vi "Channel Loop.vi"(6 "Event Based?":bool, 7 "Rate":i32=200, 8 "Index":i32, 9 "Waveform Queue":refnum<queue>, 10 "Close Event":refnum<user-event>, 11 "Channel":tag) -> (0 "error out":errorcluster)   [LabVIEW 2020]
uses:
  <vilib>/DAQmx/read.llb/DAQmx Read (Analog Wfm 1Chan NSamp).vi
  <vilib>/DAQmx/create/channels.llb/DAQmx Create Channel (AI-Voltage-Basic).vi
  <vilib>/DAQmx/configure/timing.llb/DAQmx Timing (Sample Clock).vi
  <vilib>/DAQmx/miscellaneous.llb/DAQmx Fill In Error Info.vi
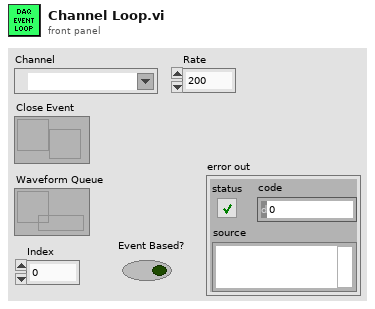
[diagram p1: front panel]
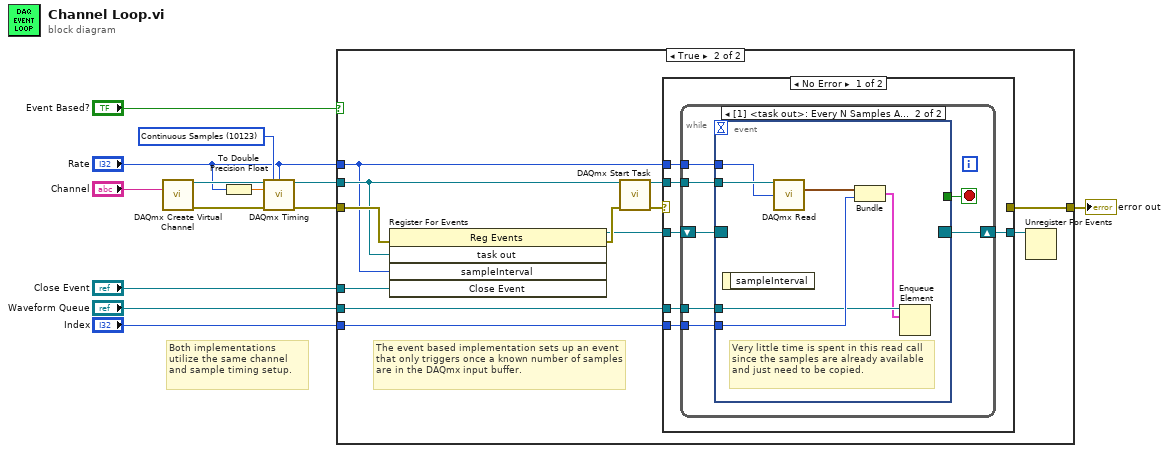
[diagram p0: block diagram]
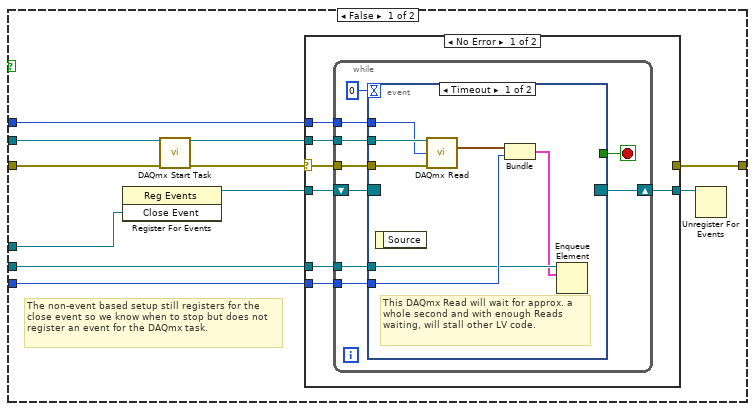
[diagram p2: hidden frame]
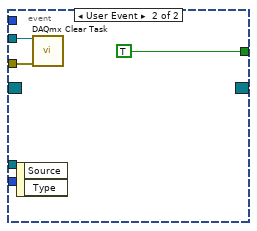
[diagram p3: hidden frame]
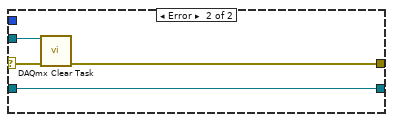
[diagram p4: hidden frame]
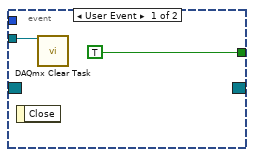
[diagram p5: hidden frame]
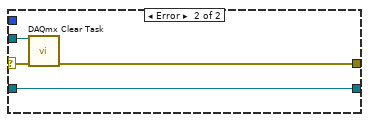
[diagram p6: hidden frame]
diagram:
  w8 = 10123 items=["Finite Samples"=10178, "Continuous Samples"=10123, "Hardware Timed Single Point"=12522] ("sample mode")
  # "Both implementations utilize the same channel and sample timing setup."
  n1 = call-poly <vilib>:"DAQmx Create Virtual Channel.vi"("physical channels"="Channel") -> ("task out"=w11:refnum<k21>, "error out"=w10:errorcluster)  [unwired: 13 in]
  n2 = To Double Precision Float(number="Rate") -> (double precision float=w9:dbl)
  n3 = call-poly <vilib>:"DAQmx Timing.vi"("task/channels in"=w11, "sample mode"=w8, "samples per channel"="Rate", "rate"=w9, "error in"=w10) -> ("task out"=w5:refnum<k21>, "error out"=w13:errorcluster)  [unwired: 9 in]
  n4 = case shown="True" "Event Based?" {
    tunnel: w13 -> [w23 w66]
    tunnel: "Close Event" -> [w22 w65]
    tunnel: "Rate" -> [w18 w55]
    tunnel: w5 -> [w24 w63]
    tunnel: "Waveform Queue" -> [w17 w59]
    tunnel: "Index" -> [w16 w58]
    tunnel: [w15 w57] -> w2
    frame False {
      # "The non-event based setup still registers for the close event so we know when to stop but does not register an event for the DAQmx task."
      n5 = register-events(w22) -> (reference out=w21:refnum<event-registration>)  [unwired: 2 in, 1 out]
      n6 = call <vilib>:"DAQmx Start Task.vi"("task/channels in"=w24, "error in"=w23) -> ("task out"=w19:refnum<k21>, "error out"=w20:errorcluster)  [unwired: 12 in]
      n7 = case shown="No Error" w20 {
        selector: w20 -> [w30 w53]
        tunnel: w21 -> [w31 w54]
        tunnel: w19 -> [w29 w52]
        tunnel: w18 -> [w28 _]
        tunnel: w17 -> [w27 _]
        tunnel: w16 -> [w26 _]
        tunnel: [w25 w54] -> w14
        tunnel: [_ w51] -> w15
        frame No Error {
          n8 = while {
            shift-right: [w38] -> w25
            shift-left: w31 -> [w39]
            tunnel: w30 -> [w36]
            tunnel: w29 -> [w37]
            tunnel: w28 -> [w35]
            tunnel: w27 -> [w33]
            tunnel: w26 -> [w32]
            stop <- w34 stop-if-true
            n9 = event shown="[0] Timeout" {
              selector: w39 -> [_ _]
              dyn-events: [_ _] -> w38
              timeout: 0 -> [_ _]
              tunnel: w37 -> [w47 w50]
              tunnel: w36 -> [w46 w49]
              tunnel: w35 -> [w45 _]
              tunnel: [_ TRUE] -> w34
              tunnel: w33 -> [w42 _]
              tunnel: w32 -> [w43 _]
              event Timeout {
                # "This DAQmx Read will wait for approx. a whole second and with enough Reads waiting, will stall other LV code."
                n10 = event-data() -> ()  [unwired: 1 in, 1 out]
                n11 = call-poly <vilib>:"DAQmx Read.vi"("task/channels in"=w47, "number of samples per channel"=w45, "error in"=w46) -> ("data"=w44:waveform(dbl))  [unwired: 10 in, 2 out]
                n12 = Bundle("data"=w44, "Index"=w43) -> (w41:cluster{"data":waveform(dbl), "Index":i32})  [unwired: 1 in]
                n13 = Enqueue Element(queue=w42, element=w41) -> ()  [unwired: 2 in, 3 out]
              }
              event User Event {
                n14 = event-data() -> ()  [unwired: 1 in, 2 out]
                n15 = call <vilib>:"DAQmx Clear Task.vi"("task in"=w50, "error in"=w49) -> ()  [unwired: 13 in, 1 out]
              }
            }
          }
        }
        frame Error {
          n16 = call <vilib>:"DAQmx Clear Task.vi"("task in"=w52, "error in"=w53) -> ("error out"=w51:errorcluster)  [unwired: 13 in]
        }
      }
      n17 = Unregister For Events(event registration refnum=w14) -> ()  [unwired: 1 in, 1 out]
    }
    frame True {
      # "The event based implementation sets up an event that only triggers once a known number of samples are in the DAQmx input buffer."
      n18 = register-events(error in=w66, w63, w55, w65) -> (reference out=w60:refnum<event-registration>, error out=w64:errorcluster)  [unwired: 1 in]
      n19 = call <vilib>:"DAQmx Start Task.vi"("task/channels in"=w63, "error in"=w64) -> ("task out"=w62:refnum<k21>, "error out"=w61:errorcluster)  [unwired: 12 in]
      n20 = case shown="No Error" w61 {
        selector: w61 -> [_ w90]
        tunnel: w62 -> [w71 w91]
        tunnel: w60 -> [w72 w88]
        tunnel: w59 -> [w70 _]
        tunnel: w58 -> [w69 _]
        tunnel: [_ w89] -> w57
        tunnel: [w68 w88] -> w56
        tunnel: w55 -> [w67 _]
        frame No Error {
          n21 = while {
            shift-right: [w78] -> w68
            shift-left: w72 -> [w79]
            tunnel: w71 -> [w76]
            tunnel: w70 -> [w75]
            tunnel: w69 -> [w74]
            tunnel: w67 -> [w73]
            stop <- w77 stop-if-true
            n22 = event shown="[1] <task out>: Every N Samples Acquired into Buffer" {
              selector: w79 -> [_ _]
              dyn-events: [_ _] -> w78
              timeout: _ -> [_ _]
              tunnel: [TRUE _] -> w77
              tunnel: w76 -> [w80 w87]
              tunnel: w75 -> [_ w84]
              tunnel: w74 -> [_ w86]
              tunnel: w73 -> [_ w82]
              event User Event {
                n23 = event-data() -> ()  [unwired: 1 in, 1 out]
                n24 = call <vilib>:"DAQmx Clear Task.vi"("task in"=w80) -> ()  [unwired: 14 in, 1 out]
              }
              event Every N Samples Acquired into Buffer {
                # "Very little time is spent in this read call since the samples are already available and just need to be copied."
                n25 = event-data() -> ()  [unwired: 1 in, 1 out]
                n26 = call-poly <vilib>:"DAQmx Read.vi"("task/channels in"=w87, "number of samples per channel"=w82) -> ("data"=w85:waveform(dbl))  [unwired: 11 in, 2 out]
                n27 = Bundle("data"=w85, "Index"=w86) -> (w83:cluster{"data":waveform(dbl), "Index":i32})  [unwired: 1 in]
                n28 = Enqueue Element(queue=w84, element=w83) -> ()  [unwired: 2 in, 3 out]
              }
            }
          }
        }
        frame Error {
          n29 = call <vilib>:"DAQmx Clear Task.vi"("task in"=w91, "error in"=w90) -> ("error out"=w89:errorcluster)  [unwired: 13 in]
        }
      }
      n30 = Unregister For Events(event registration refnum=w56) -> ()  [unwired: 1 in, 1 out]
    }
  }
  "error out" <- w2
